vi "test_Util_All.vi"(8 "error in (no error)":errorcluster) -> (0 "error out":errorcluster, 3 "Test Passed":bool)   [LabVIEW 2019]
panel:
  out "April Tag Utils Passed":bool
  out "Xform Test Passed":bool
  out "Dist Test Passed":bool
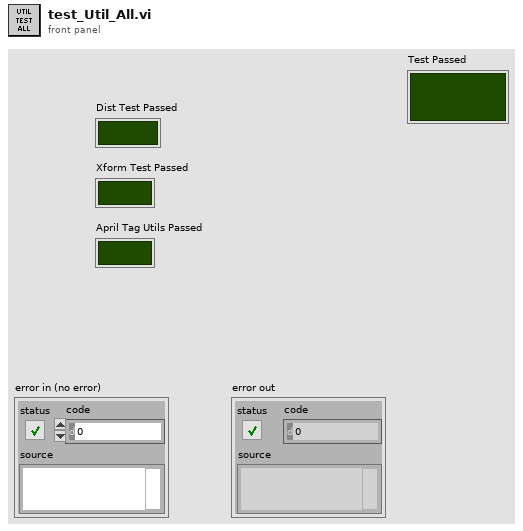
[diagram p1: front panel]
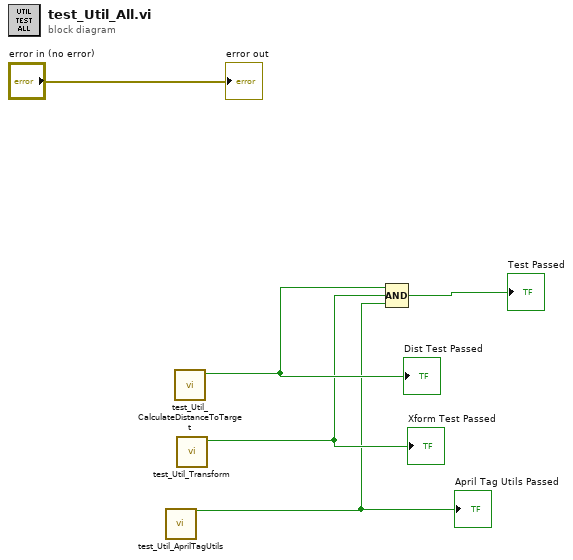
[diagram p0: block diagram]
diagram:
  n1 = call "test_Util_AprilTagUtils.vi"() -> ("Test Passed"=w1:bool)  [unwired: 10 in, 1 out]
  "April Tag Utils Passed" <- w1
  n2 = call "test_Util_CalculateDistanceToTarget.vi"() -> ("Test Passed"=w3:bool)  [unwired: 10 in, 1 out]
  "Dist Test Passed" <- w3
  n3 = call "test_Util_Transform.vi"() -> ("Test Passed"=w2:bool)  [unwired: 10 in, 1 out]
  "Xform Test Passed" <- w2
  n4 = Compound Arithmetic op=AND(w3, w2, w1) -> (→"Test Passed":bool)
  "error out" <- "error in (no error)"
